vi "TestExec.Net Use Config - Dialog.vi"(11 "Config Dir":path=path "C:/MTE/Knuckles Function Test/Config") -> (1 "OK":bool)   [LabVIEW 2024]
uses:
  <vilib>/KATE/Files/File Utils.lvlib
  <vilib>/KATE/Encryption/Encryption.lvlib
panel:
  out "Tab Control":enum32{"Input", "Dialog", "Output"}(tab)=enum."Dialog"
  in  "Test":bool
  in  "Net Use Items":T1(array[cluster])
  in  "Cancel Button":bool
  in  "OK Button":bool
  out "Net Use CSV File":path
  out "Table Control":string[][](table)
  # "Net Use Setup"
  # "domain\\user"
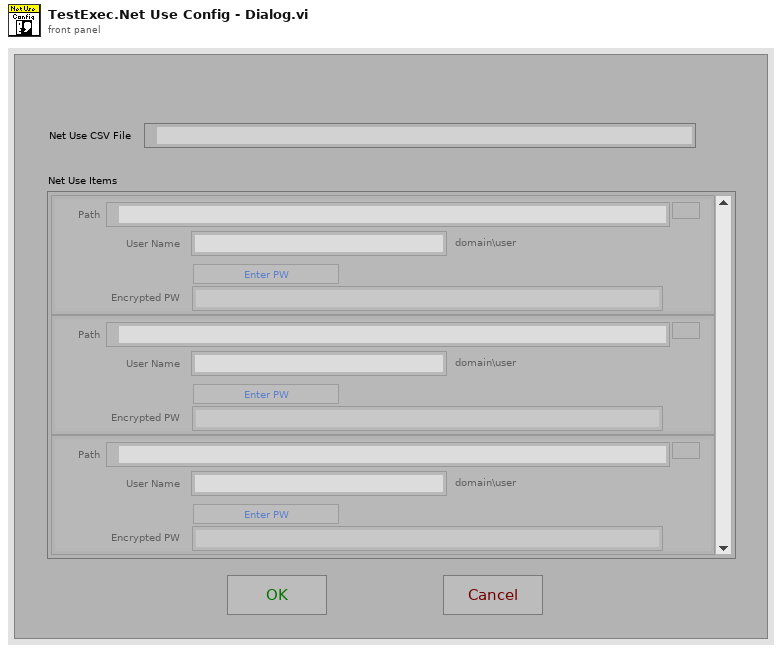
[diagram p1: front panel]
types:
  T1 = cluster{"Path":path, "User Name":string, "EncPW":string, "EnterPW":bool}[]
  T2 = cluster{"Path":path, "User Name":string, "Encrypted Password":string, "EnterPW":bool}
  T3 = enum16{"open", "replace", "create", "open or create", "replace or create", "replace or create with confirmation"}
  T4 = enum32{"Invalid", "Standard", "Closed", "Hidden", "Minimized", "Maximized"}
  T5 = cluster{"Path":path, "User Name":string, "EncPW":string, "EnterPW":bool}
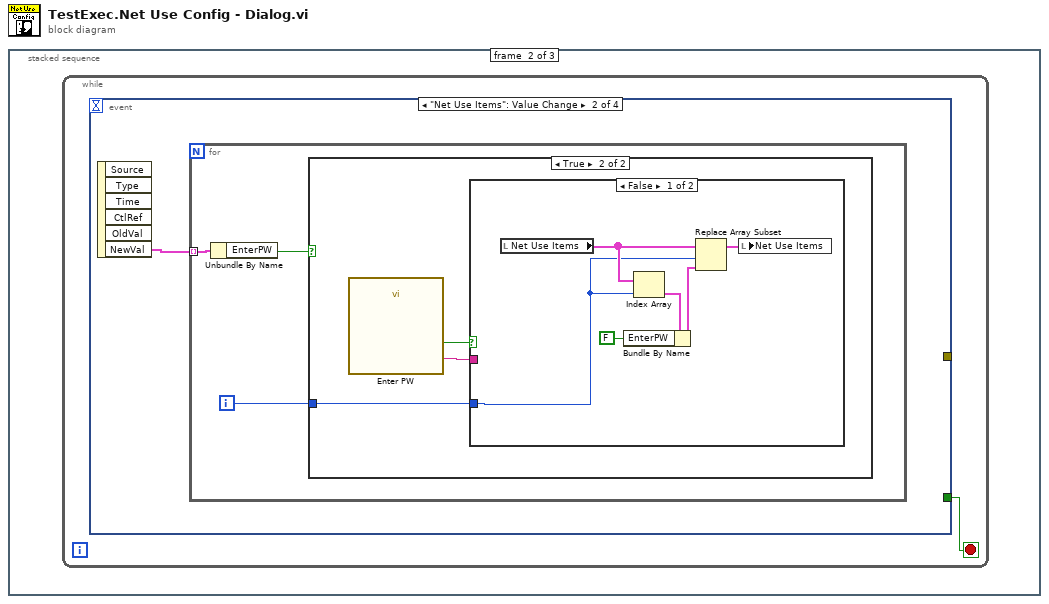
[diagram p0: block diagram]
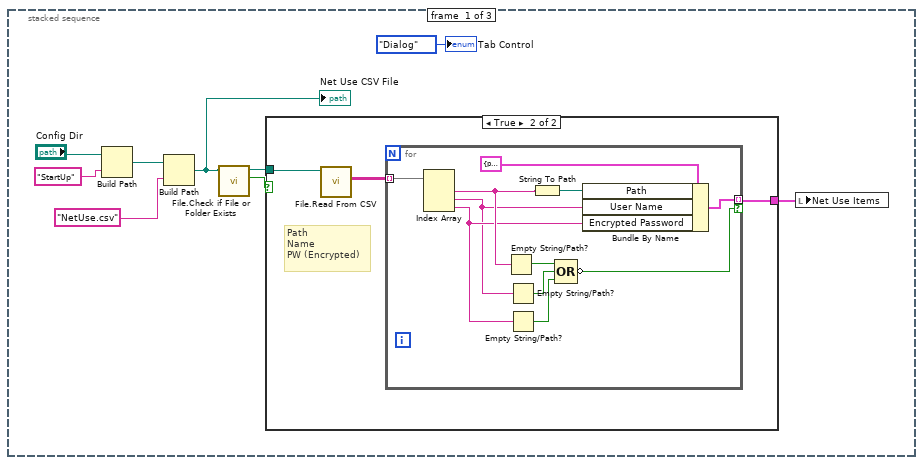
[diagram p2: hidden frame]
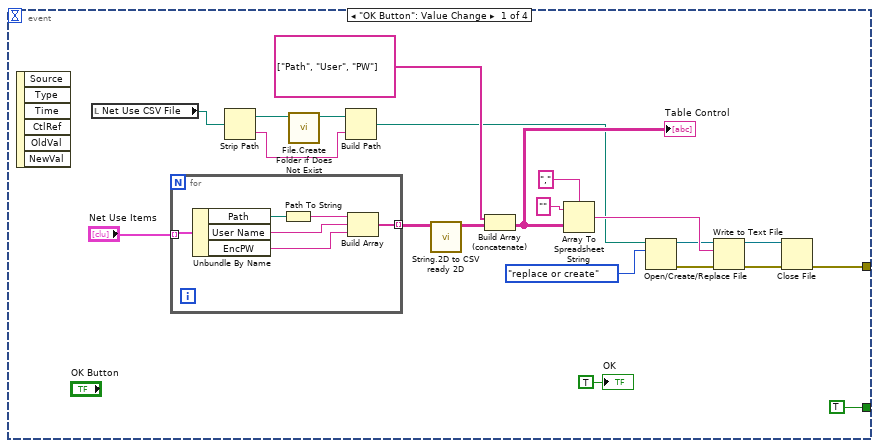
[diagram p4: hidden frame]
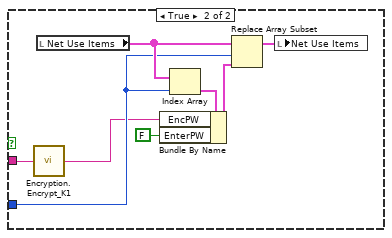
[diagram p6: hidden frame]
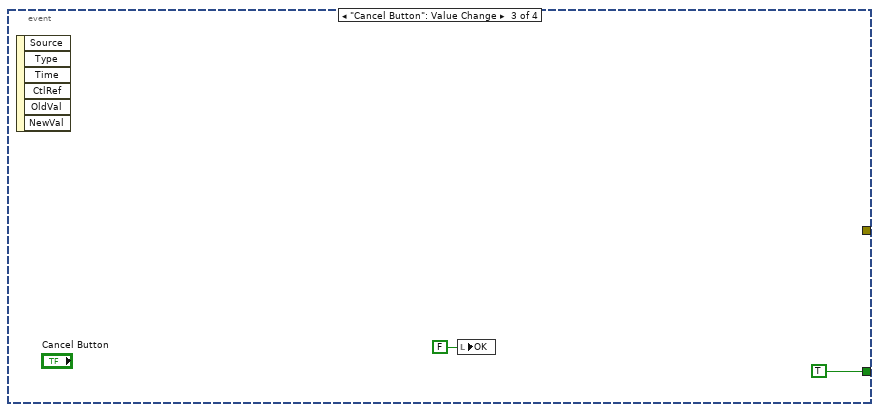
[diagram p7: hidden frame]
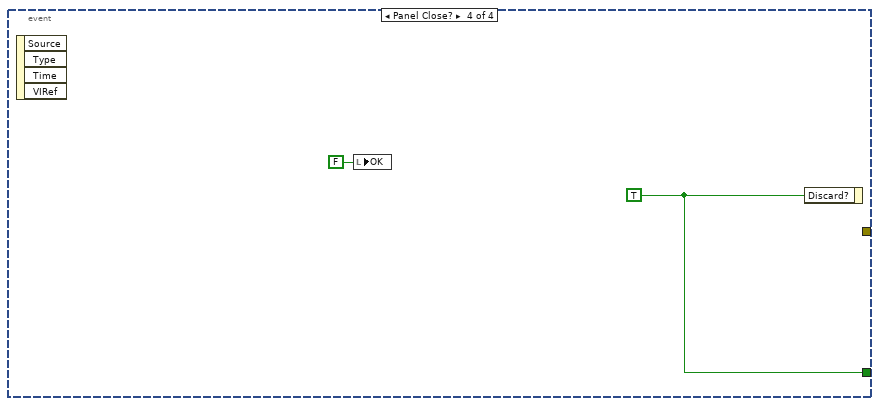
[diagram p8: hidden frame]
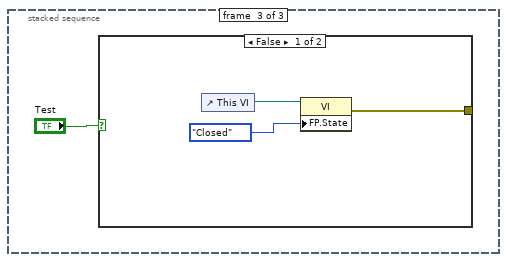
[diagram p9: hidden frame]
diagram:
  n1 = stacked-sequence {
    frame #0 {
      n2 = Build Path(base path="Config Dir", name or relative path="StartUp") -> (appended path=w7:path)
      n3 = Build Path(base path=w7, name or relative path="NetUse.csv") -> (appended path=w5:path)
      "Net Use CSV File" <- w5
      n4 = call <vilib>:"File.Check if File or Folder Exists.vi"("Path"=w5) -> ("Exists"=w4:bool, "Dup Path"=w3:path)  [unwired: 6 in, 3 out]
      n5 = case shown="True" w4 {
        tunnel: w3 -> [_ w11]
        tunnel: [_ w10] -> w2
        frame False {
        }
        frame True {
          # "Path\nName\nPW (Encrypted)"
          n6 = call <vilib>:"File.Read From CSV.vi"("File"=w11) -> ("Data"=w12:string[][])  [unwired: 8 in, 2 out]
          n7 = for {
            tunnel: w12 -> [w23] mode=indexing
            tunnel: [w15] -> w10 mode=indexing if=w19
            n8 = Index Array(array=w23) -> (element #1=w16:string, element #2=w13:string, element #3=w14:string)  [unwired: 3 in]
            n9 = Empty String/Path?(string/path=w16) -> (empty?=w22:bool)
            n10 = Empty String/Path?(string/path=w13) -> (empty?=w21:bool)
            n11 = Empty String/Path?(string/path=w14) -> (empty?=w20:bool)
            n12 = String To Path(string=w16) -> (path=w17:path)
            n13 = Compound Arithmetic op=OR(w22, w21, w20) -> (invert w19:bool)
            n14 = Bundle By Name(cluster=T2 {"Path"=path "", "User Name"="", "Encrypted Password"="", "EnterPW"=FALSE} ("Cluster"), "Path"=w17, "User Name"=w13, "Encrypted Password"=w14) -> (w15:T2)
          }
        }
      }
      n15 = local write "Net Use Items"(w2) -> ()
      "Tab Control" <- enum32{"Input", "Dialog", "Output"}."Dialog" ("Tab Control")
    }
    frame #1 {
      n16 = while {
        stop <- w24 stop-if-true
        n17 = event shown="[1] \"Net Use Items\": Value Change" {
          selector: _ -> [_ _ _ _]
          dyn-events: _ -> [_ _ _ _]
          timeout: _ -> [_ _ _ _]
          tunnel: [TRUE _ TRUE w75] -> w24
          tunnel: [w26 _ _ _] -> _
          event "OK Button": Value Change {
            n18 = event-data() -> ()  [unwired: 1 in, 6 out]
            n19 = local read "Net Use CSV File"() -> (w35:path)
            n20 = for {
              tunnel: "Net Use Items" -> [w51] mode=indexing
              tunnel: [w46] -> w43 mode=indexing
              n21 = Unbundle By Name(w51) -> ("Path"=w50:path, "User Name"=w48:string, "EncPW"=w47:string)
              n22 = Path To String(path=w50) -> (string=w49:string)
              n23 = Build Array(w49, w48, w47) -> (w46:string[])
            }
            n24 = Strip Path(path=w35) -> (stripped path=w34:path, name=w32:string)
            n25 = call <vilib>:"File.Create Folder if Does Not Exist.vi"("Path"=w34) -> ("Dup Path"=w33:path)  [unwired: 8 in, 2 out]
            n26 = Build Path(base path=w33, name or relative path=w32) -> (appended path=w31:path)
            n27 = call "String.2D to CSV ready 2D.vi"("2D In"=w43) -> ("2D In Out"=w38:string[][])  [unwired: 10 in]
            n28 = Build Array (concatenate)(string[] ["Path", "User", "PW"], w38) -> (w36:string[][])
            "Table Control" <- w36
            n29 = Array To Spreadsheet String(delimiter (Tab)=",", array=w36, 3:"" ("format string")) -> (spreadsheet string=w40:string)
            n30 = Open/Create/Replace File(file path (use dialog)=w31, operation (0:open)=T3."replace or create") -> (refnum out=w30:refnum<file>, error out=w28:errorcluster)  [unwired: 4 in, 1 out]
            n31 = Write to Text File(file (use dialog)=w30, text=w40, error in=w28) -> (refnum out=w29:refnum<file>, error out=w27:errorcluster)  [unwired: 1 in, 1 out]
            n32 = Close File(refnum=w29, error in=w27) -> (error out=w26:errorcluster)  [unwired: 1 out]
            "OK" <- TRUE ("OK")
          }
          event "Net Use Items": Value Change {
            n33 = event-data() -> ("NewVal"=w52:T1)  [unwired: 1 in, 5 out]
            n34 = for {
              tunnel: w52 -> [w55] mode=indexing
              i -> [w54]
              n35 = Unbundle By Name(w55) -> ("EnterPW"=w53:bool)
              n36 = case shown="True" w53 {
                tunnel: w54 -> [_ w58]
                frame False {
                }
                frame True {
                  n37 = call "Enter PW"() -> ("PW"=w56:string, "OK"=w57:bool)  [unwired: 17 in, 1 out]
                  n38 = case shown="False" w57 {
                    tunnel: w58 -> [w59 w70]
                    tunnel: w56 -> [_ w67]
                    frame False {
                      n39 = local read "Net Use Items"() -> (w63:T1)
                      n40 = Index Array(array=w63, index=w59) -> (element=w62:T5)
                      n41 = Bundle By Name(cluster=w62, "EnterPW"=FALSE) -> (w61:T5)
                      n42 = Replace Array Subset(array=w63, new element=w61, index=w59) -> (w64:T1)
                      n43 = local write "Net Use Items"(w64) -> ()
                    }
                    frame True {
                      n44 = call <vilib>:"Encryption.Encrypt_K1.vi"("String"=w67) -> ("Encrypted String"=w66:string)
                      n45 = local read "Net Use Items"() -> (w71:T1)
                      n46 = Index Array(array=w71, index=w70) -> (element=w69:T5)
                      n47 = Bundle By Name(cluster=w69, "EncPW"=w66, "EnterPW"=FALSE) -> (w68:T5)
                      n48 = Replace Array Subset(array=w71, new element=w68, index=w70) -> (w72:T1)
                      n49 = local write "Net Use Items"(w72) -> ()
                    }
                  }
                }
              }
            }
          }
          event "Cancel Button": Value Change {
            n50 = event-data() -> ()  [unwired: 1 in, 6 out]
            n51 = local write "OK"(FALSE ("OK")) -> ()
          }
          event Panel Close? {
            w75 = TRUE ("Discard?")
            n52 = event-data() -> ()  [unwired: 1 in, 4 out]
            n53 = local write "OK"(FALSE ("OK")) -> ()
            n54 = event-data("Discard?"=w75) -> ()  [unwired: 1 in, 1 out]
          }
        }
      }
    }
    frame #2 {
      n55 = case shown="False" "Test" {
        tunnel: [w78 _] -> _
        frame False {
          n56 = control-ref of="This VI"() -> (w80:refnum<vi>)
          n57 = property class="VI"(reference=w80, "FP.State"=T4."Closed" ("Front Panel Window:State")) -> (error out=w78:errorcluster)  [unwired: 1 in, 1 out]
        }
        frame True {
        }
      }
    }
  }
